vi "CavityConstanstToFIFO.vi"(0 "w12":dbl format="%#_12g", 5 "R1":dbl, 7 "w1":dbl, 9 "Q1":dbl, 11 "K1":dbl, 12 "S":dbl) -> (4 "FIFO array":u64[](array[numeric]))   [LabVIEW 2013]
uses:
  FPGA/fpga_settings.ctl
  <vilib>/rvi/FXPMathLib/FxpInterpret/XNode/nifxpmath_Interpret.xnode
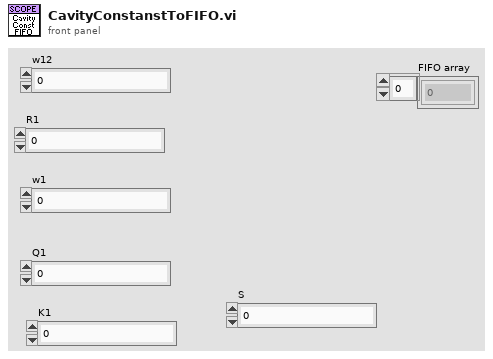
[diagram p1: front panel]
types:
  T1 = typedef "fpga_settings.ctl" = enum16{"Feedback Enable", "New FIR coeffs", "FIR shift", "Enable filter", "Set Downsample", "Downsample", "CIC Gain", "Record length", "Trigger samples", "Quiet time", "a_am", "b_am", "Use fixed delay", "fixed sin_fi", "fixed cos_fi", "Ki*Tau", "Kp", "Kd_Tau", "Fi_start", "Fi_delta", "DC_offs 0", "DC_offs 1", "DC_offs 2", "DC_offs 3", "Ki*Tau am", "Kp am", "Kd_Tau am", "Feedback AM", "Trigger delay", "Feedback delay", "Setpoint enable", "Beam enable", "Samples to acquire", "Cavity Enable", "Cavity C1", "Cavity C2", "Cavity C3", "Cavity C4", "Cavity C5"}
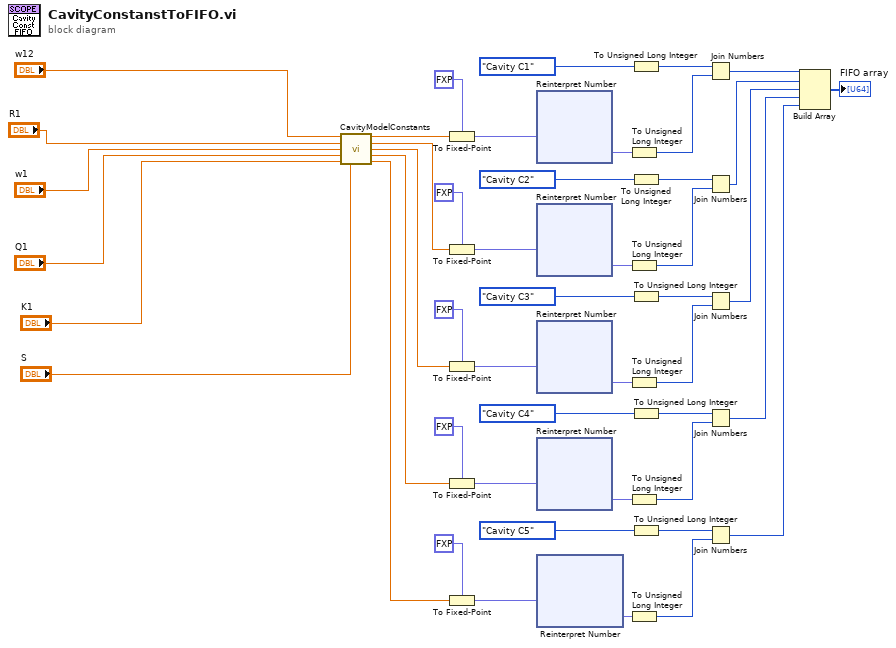
[diagram p0: block diagram]
diagram:
  n1 = call "CavityModelConstants.vi"("w12"="w12", "R1"="R1", "w1"="w1", "Q1"="Q1", "K1"="K1", "S"="S") -> ("C1"=w45:dbl, "C2"=w15:dbl, "C3"=w13:dbl, "C4"=w14:dbl, "C5"=w12:dbl)  [unwired: 5 in]
  n2 = To Fixed-Point(fixed-point type=fxp<+/-,32,1> 0.0 ("x"), number=w45) -> (fixed-point=w47:fxp<+/-,32,1>)
  n3 = To Fixed-Point(fixed-point type=fxp<+/-,32,3> 0.0 ("x"), number=w15) -> (fixed-point=w34:fxp<+/-,32,3>)
  n4 = To Fixed-Point(fixed-point type=fxp<+/-,32,3> 0.0 ("x"), number=w13) -> (fixed-point=w33:fxp<+/-,32,3>)
  n5 = To Fixed-Point(fixed-point type=fxp<+/-,32,1> 0.0 ("x"), number=w14) -> (fixed-point=w22:fxp<+/-,32,1>)
  n6 = To Fixed-Point(fixed-point type=fxp<+/-,32,-32> 0.0 ("x"), number=w12) -> (fixed-point=w21:fxp<+/-,32,-32>)
  n7 = xnode "Reinterpret Number"("x"=w47) -> ("y"=w41:fxp<+,32,32>)
  n8 = xnode "Reinterpret Number"("x"=w34) -> ("y"=w39:fxp<+,32,32>)
  n9 = xnode "Reinterpret Number"("x"=w33) -> ("y"=w28:fxp<+,32,32>)
  n10 = xnode "Reinterpret Number"("x"=w22) -> ("y"=w27:fxp<+,32,32>)
  n11 = xnode "Reinterpret Number"("x"=w21) -> ("y"=w16:fxp<+,32,32>)
  n12 = To Unsigned Long Integer(number=w41) -> (unsigned 32bit integer=w44:u32)
  n13 = To Unsigned Long Integer(number=w39) -> (unsigned 32bit integer=w36:u32)
  n14 = To Unsigned Long Integer(number=w28) -> (unsigned 32bit integer=w31:u32)
  n15 = To Unsigned Long Integer(number=w27) -> (unsigned 32bit integer=w24:u32)
  n16 = To Unsigned Long Integer(number=w16) -> (unsigned 32bit integer=w19:u32)
  n17 = To Unsigned Long Integer(number=fpga_settings."Cavity C1" ("FPGA Setting")) -> (unsigned 32bit integer=w42:u32)
  n18 = To Unsigned Long Integer(number=fpga_settings."Cavity C2" ("FPGA Setting")) -> (unsigned 32bit integer=w38:u32)
  n19 = To Unsigned Long Integer(number=fpga_settings."Cavity C3" ("FPGA Setting")) -> (unsigned 32bit integer=w29:u32)
  n20 = To Unsigned Long Integer(number=fpga_settings."Cavity C4" ("FPGA Setting")) -> (unsigned 32bit integer=w26:u32)
  n21 = To Unsigned Long Integer(number=fpga_settings."Cavity C5" ("FPGA Setting")) -> (unsigned 32bit integer=w17:u32)
  n22 = Join Numbers(hi=w42, lo=w44) -> ((hi.lo)=w40:u64)
  n23 = Join Numbers(hi=w38, lo=w36) -> ((hi.lo)=w11:u64)
  n24 = Join Numbers(hi=w29, lo=w31) -> ((hi.lo)=w10:u64)
  n25 = Join Numbers(hi=w26, lo=w24) -> ((hi.lo)=w9:u64)
  n26 = Join Numbers(hi=w17, lo=w19) -> ((hi.lo)=w8:u64)
  n27 = Build Array(w40, w11, w10, w9, w8) -> (→"FIFO array":u64[])
